vi "BIO_push.vi"(8 "error in (no error)":errorcluster, 10 "New BIO":refnum<class "BIO.lvclass">, 11 "BIO in":refnum<class "BIO.lvclass">) -> (0 "error out":errorcluster, 3 "BIO out":refnum<class "BIO.lvclass">)   [LabVIEW 2013, in "OpenSSL Socket.lvlib" / "BIO.lvclass"]
uses:
  BIO.lvclass
  SSL-Lib/SSL-Lib.lvclass/SSL-Lib.ctl
  BIO.lvclass/BIO.ctl
  Read Handle.vi
  SSL-Lib/Read Crypto Library Path.vi
  SSL-Lib/SSL-Lib.lvclass
panel:
  out "BIO":u64
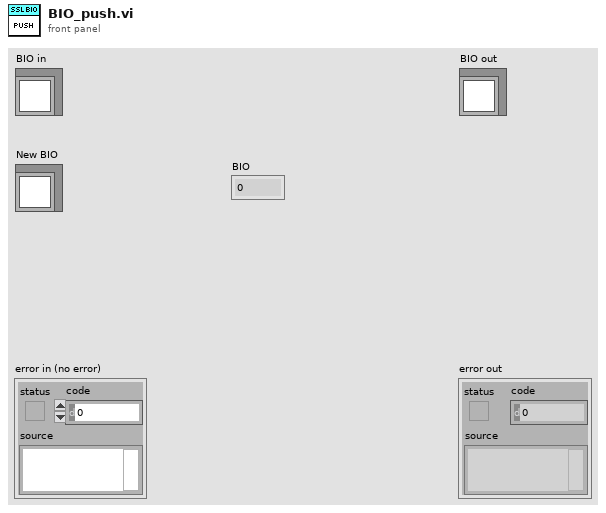
[diagram p1: front panel]
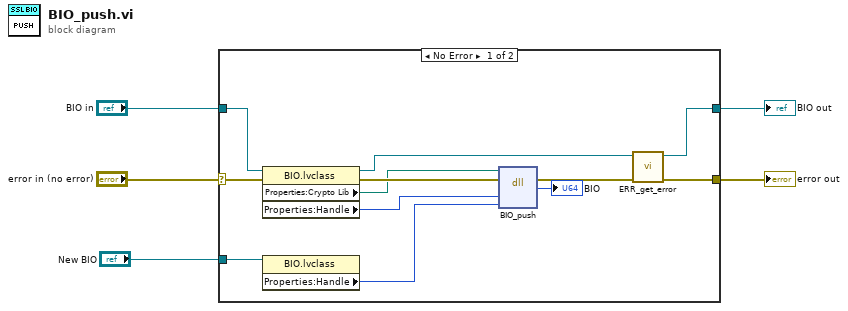
[diagram p0: block diagram]
diagram:
  n1 = case shown="No Error" "error in (no error)" {
    selector: "error in (no error)" -> [w17 w19]
    tunnel: [w10 w19] -> w4
    tunnel: [w8 w18] -> w2
    tunnel: "BIO in" -> [w14 w18]
    tunnel: "New BIO" -> [w11 _]
    frame No Error {
      n2 = property class="BIO.lvclass"(reference=w14, error in=w17) -> (reference out=w9:refnum<class "BIO.lvclass">, error out=w15:errorcluster, "Properties:Crypto Lib"=w13:path, "Properties:Handle"=w12:u64)
      n3 = property class="BIO.lvclass"(reference=w11) -> ("Properties:Handle"=w7:u64)  [unwired: 1 in, 2 out]
      n4 = dll-call lib="C:/Program Files (x86)/National Instruments/Shared/nissl/NIlibeay32.dll" fn="BIO_push"(path in=w13, error in=w15, "BIO"=w12, "appendBIO"=w7) -> (error out=w16:errorcluster, "BIO"=→"BIO":u64)  [unwired: 3 in, 1 out]
      n5 = call "ERR_get_error.vi"("error in (no error)"=w16, "SSL-Lib in"=w9) -> ("error out"=w10:errorcluster, "SSL-Lib out"=w8:refnum<class "BIO.lvclass">)  [unwired: 8 in]
    }
    frame Error {
    }
  }
  "error out" <- w4
  "BIO out" <- w2
